vi "DI Check.vi"(5 "Boolean in":bool, 6 "millisecond timer value":u32, 7 "DI value in":bool[](array[boolean]), 8 "error in (no error)":errorcluster, 9 "DI Index":i32[](array[numeric]), 10 "Cluster":T1, 11 "DI read":bool[](array[boolean])=[FALSE, FALSE, FALSE, FALSE, FALSE, FALSE, FALSE]) -> (1 "DI value out":bool[](array[boolean]), 2 "Abort Seq":bool, 3 "Boolean out":bool)   [LabVIEW 2022 SP3]
uses:
  <vilib>/Platform/TimedLoop/XDataNode/wakeup.ctl
  <vilib>/Platform/TimedLoop/XDataNode/XDNodeRunTimeDep.lvlib
  <vilib>/Platform/TimedLoop/XDataNode/nitl_modes.ctl
  <vilib>/Platform/TimedLoop/XDataNode/timing_clust.ctl
  <vilib>/platform/TimedLoop/XDataNode/XDataNode.xnode
  RT Sub VI's/RT Global.vi
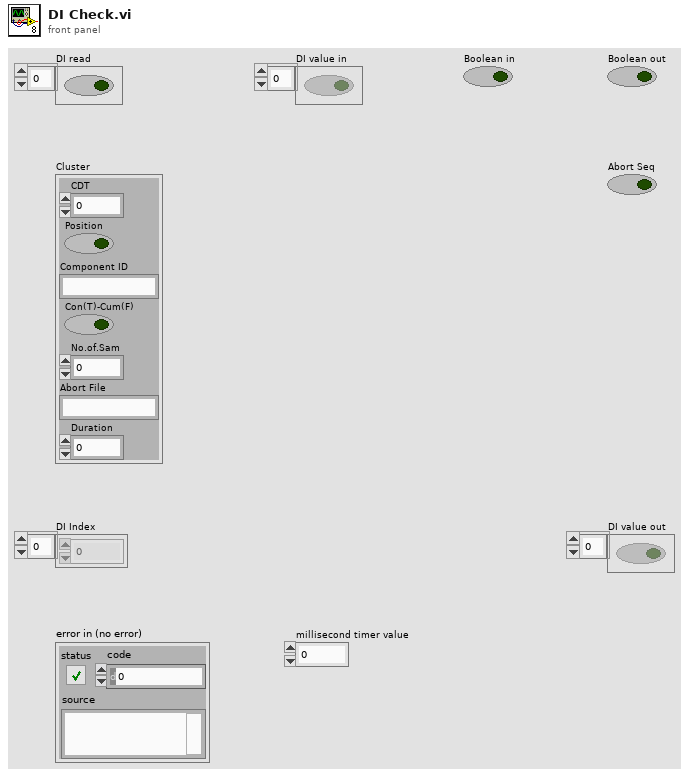
[diagram p1: front panel]
types:
  T1 = cluster{"CDT":dbl, "Position":bool, "Component ID":string, "Con(T)-Cum(F)":bool, "No.of.Sam":dbl, "Abort File":string, "Duration":u32}
  T2 = typedef "XDNodeRunTimeDep.lvlib/timing_clust.ctl" = cluster{"Expected End [f-1]":u64, "Actual End [f-1]":u64, "Finished Late? [f-1]":bool, "Expected End [i-1]":u64, "Actual End [i-1]":u64, "Finished Late? [i-1]":bool, "Expected Start [i]":u64, "Actual Start [i]":u64, "Expected Start [f]":u64, "Actual Start [f]":u64, "Source Name":string, "Structure Name":string, "Period":i64, "Deadline":i64, "Offset":i64, "Start":i64, "Priority":i32, "Timeout":i32, "Mode":T3, "Wakeup Reason":T4, "Error":errorcluster, "Source Type":string, "Secondary Source Type":string, "Global End Time":u64, "Global Start Time":u64, "Frame Duration":u64, "Iteration Duration":u64, "Assigned CPU":i32, "I/O Scan Engine Mode":u32}
  T3 = typedef "XDNodeRunTimeDep.lvlib/nitl_modes.ctl" = enum32{"No Change", "Process missed periods, maintain original phase", "Discard missed periods, maintain original phase", "Process missed periods, ignore original phase", "Discard missed periods, ignore original phase"}
  T4 = typedef "XDNodeRunTimeDep.lvlib/wakeup.ctl" = enum32{"Normal", "Aborted", "Asynchronous wakeup", "Timing source error", "Timed loop error", "Timeout"}
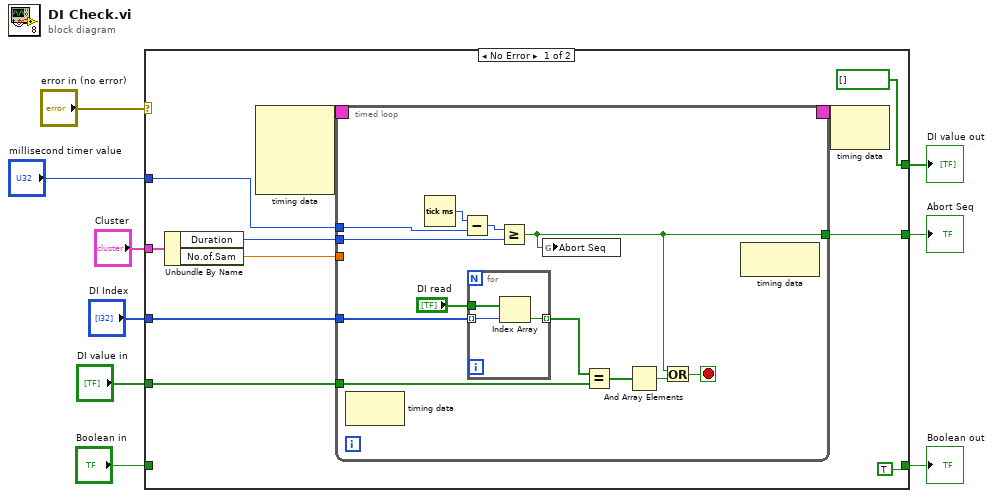
[diagram p0: block diagram]
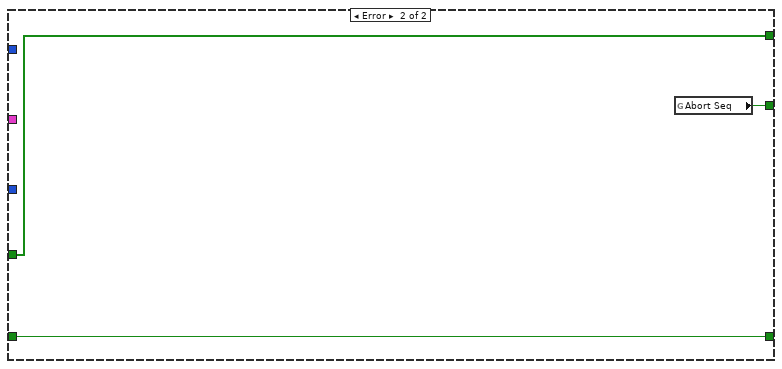
[diagram p2: hidden frame]
diagram:
  n1 = case shown="No Error" "error in (no error)" {
    tunnel: "DI value in" -> [w19 w42]
    tunnel: [bool[] [] ("DO value") w42] -> w3
    tunnel: [w17 w41] -> w7
    tunnel: "DI Index" -> [w20 _]
    tunnel: "Boolean in" -> [_ w40]
    tunnel: [TRUE ("Boolean in") w40] -> w6
    tunnel: "millisecond timer value" -> [w18 _]
    tunnel: "Cluster" -> [w15 _]
    frame No Error {
      n2 = Unbundle By Name(w15) -> ("Duration"=w14:u32, "No.of.Sam"=w11:dbl)
      n3 = node-c288() -> (w13:T2)  [unwired: 4 in]
      n4 = timed-loop {
        tunnel: w20 -> [w31]
        tunnel: w19 -> [w29]
        tunnel: w18 -> [w26]
        tunnel: w14 -> [w24]
        tunnel: [w21] -> w17
        timing: w13 -> [_]
        timing-out: [_] -> w12
        tunnel: w11 -> [_]
        stop <- w22 stop-if-true
        n5 = node-c288() -> ()  [unwired: 1 in, 1 out]
        n6 = Tick Count (ms)() -> (millisecond timer value=w27:u32)
        n7 = Subtract(x=w27, y=w26) -> (x-y=w25:u32)
        n8 = for {
          tunnel: "DI read" -> [w37]
          tunnel: w31 -> [w36] mode=indexing
          tunnel: [w35] -> w30 mode=indexing
          n9 = Index Array(array=w37, index=w36) -> (element=w35:bool)
        }
        n10 = Greater Or Equal?(x=w25, y=w24) -> (x >= y?=w21:bool)
        n11 = global write "RT Global.vi" "Abort Seq"(w21) -> ()
        n12 = Equal?(x=w30, y=w29) -> (x = y?=w28:bool[])
        n13 = And Array Elements(Boolean array=w28) -> (logical AND=w23:bool)
        n14 = Or(x=w21, y=w23) -> (x .or. y?=w22:bool)
        n15 = node-c288() -> ()  [unwired: 1 in, 1 out]
      }
      n16 = node-c288(w12) -> ()  [unwired: 1 out]
    }
    frame Error {
      n17 = global read "RT Global.vi" "Abort Seq"() -> (w41:bool)
    }
  }
  "Abort Seq" <- w7
  "Boolean out" <- w6
  "DI value out" <- w3
